vi "Get Value from JSON Text with Parameter.vi"(8 "error in (no error)":errorcluster, 10 "Parameter":string, 11 "JSON Configuration File (.json)":path=path "C:/Users/chericks/Desktop/JSONtest/labview-grpc-query-server/jsontestfile2.json") -> (0 "error out":errorcluster, 2 "Value":string="6")   [LabVIEW 2019]
panel:
  in  "Parameter List (for unit testing)":string[](array[string])=["GETCONF=SMUResourceName", "GETCONF=SMUChannels", "GETCONF=SMUSourceMode_Sequence", "GETCONF=SMUOutputFunction_DCCurrent", "GETCONF=SMUSourceTransientResponse_Fast", "GETCONF=SMUCurrent", "GETCONF=SMUCurrentLevelRange", "GETCONF=SMUMeasurementSense_Local", "GETCONF=SMUMeasurementApertureTime", "GETCONF=SMUSourceAdvancedSourceDelay", "GETCONF=SMUVoltage", "GETCONF=SMUSourceAdvancedSequenceLoopCount", "GETCONF=SMUMeasurementAdvancedDCNoiseRejection_Normal", "GETCONF=SMUSequenceName", "GETCONF=SMUStep1_Source_DCCurrent_CurrentLevel", "GETCONF=SMUStep2_Measurement_ApertureTime", "GETCONF=SMUStep3_Source_Advanced_SourceDelay", "GETCONF=SMUSequenceNumberOfSteps", "GETCONF=SMUTriggerFromSwitch_StartDigitalEdge", "GETCONF=SMUTriggerFromSwitch_SequenceAdvanceDigitalEdge", "GETCONF=SMUTriggerToDMM_SourceCompleteEvent", "GETCONF=SMUTriggerToDMM_SourceCompleteEvent_Value", "GETCONF=SMUTriggerToSwitch_SequenceIterationCompleteEvent", "GETCONF=SMUTriggerToDMM_SequenceIterationCompleteEvent_Value", "GETCONF=Switch1ResourceName", "GETCONF=Switch1Topology", "GETCONF=Switch1ScanList", "GETCONF=Switch2ResourceName", "GETCONF=Switch2Topology", "GETCONF=Switch2ScanList", "GETCONF=DMMResourceName", "GETCONF=DMMFunction_DCVolts", "GETCONF=DMMResolution", "GETCONF=DMMRange", "GETCONF=DMMTriggerSource_TTL2", "GETCONF=DMMTriggerSlope_RisingEdge", "GETCONF=DMMSampleTrigger_TTL2", "GETCONF=DMMSampleCount", "GETCONF=DMMSampleTriggerSlope_RisingEdge", "GETCONF=DMMApertureTimeUnits_Seconds", "GETCONF=DMMApertureTime", "GETCONF=DMMNumberOfAverages", "GETCONF=DMMAutoZero_Off", "GETCONF=DMMADCCalibration_Off", "GETCONF=DMMSettleTime", "GETCONF=DMMControlAction_Commit", "GETCONF=ApplicationNumberOfWeldChannels"]
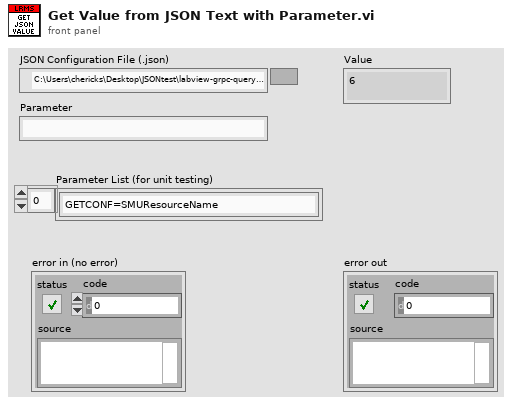
[diagram p1: front panel]
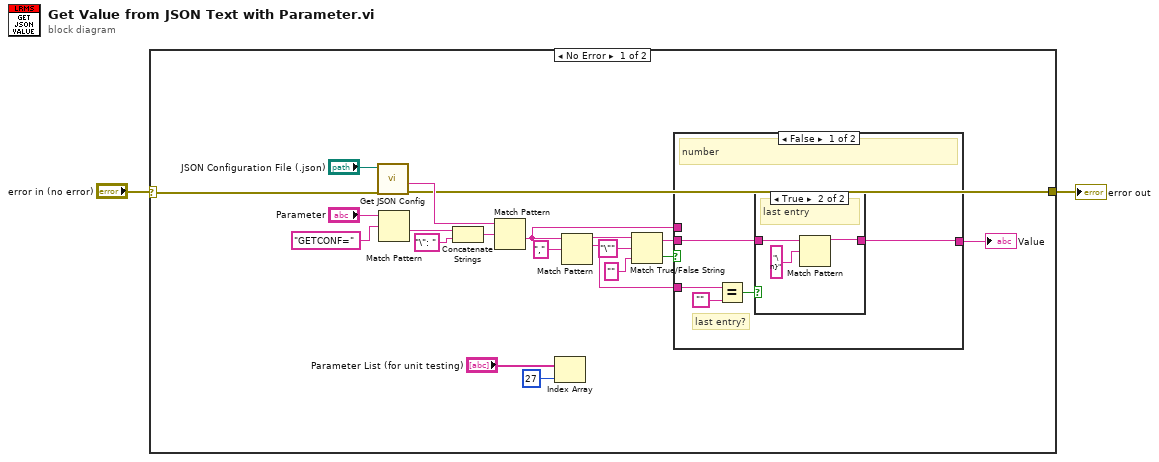
[diagram p0: block diagram]
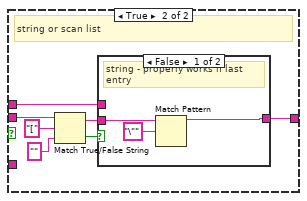
[diagram p3: hidden frame]
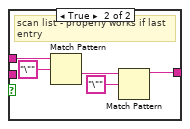
[diagram p4: hidden frame]
diagram:
  n1 = case shown="No Error" "error in (no error)" {
    selector: "error in (no error)" -> [w4 w47]
    tunnel: [w3 w47] -> w1
    frame No Error {
      n2 = call "Get JSON Config.vi"("error in (no error)"=w4, "JSON Configuration File (.json)"="JSON Configuration File (.json)") -> ("error out"=w3:errorcluster, "File Contents"=w5:string)  [unwired: 6 in, 2 out]
      n3 = Match Pattern(string="Parameter", regular expression="GETCONF=" ("default value 1")) -> (after substring=w10:string)  [unwired: 1 in, 3 out]
      n4 = Concatenate Strings(w10, "\": " ("string")) -> (w13:string)
      n5 = Match Pattern(string=w5, regular expression=w13) -> (after substring=w21:string)  [unwired: 1 in, 3 out]
      n6 = Index Array(array="Parameter List (for unit testing)", index=27) -> ()  [unwired: 1 out]
      n7 = Match Pattern(string=w21, regular expression=",") -> (before substring=w17:string, match substring=w19:string)  [unwired: 1 in, 2 out]
      n8 = Match True/False String(2:"" ("false string"), 3:"\"" ("true string"), 4:w17) -> (0:w18:bool, 1:w20:string)
      n9 = case shown="False" w18 {
        tunnel: [w23 w34] -> w9
        tunnel: w19 -> [w26 _]
        tunnel: w20 -> [w24 w38]
        tunnel: w21 -> [_ w33]
        frame False {
          # "last entry?"
          # "number"
          n10 = Equal?(x=w26, y="") -> (x = y?=w25:bool)
          n11 = case shown="True" w25 {
            tunnel: w24 -> [w28 w31]
            tunnel: [w28 w29] -> w23
            frame False {
              # "not last entry"
            }
            frame True {
              # "last entry"
              n12 = Match Pattern(string=w31, regular expression="\n}" ("string")) -> (before substring=w29:string)  [unwired: 1 in, 3 out]
            }
          }
        }
        frame True {
          # "string or scan list"
          n13 = Match True/False String(2:"" ("false string"), 3:"[" ("true string"), 4:w38) -> (0:w35:bool, 1:w32:string)
          n14 = case shown="False" w35 {
            tunnel: [w39 w42] -> w34
            tunnel: w33 -> [_ w46]
            tunnel: w32 -> [w41 _]
            frame False {
              # "string - properly works if last entry"
              n15 = Match Pattern(string=w41, regular expression="\"") -> (before substring=w39:string)  [unwired: 1 in, 3 out]
            }
            frame True {
              # "scan list - properly works if last entry"
              n16 = Match Pattern(string=w46, regular expression="\"") -> (after substring=w44:string)  [unwired: 1 in, 3 out]
              n17 = Match Pattern(string=w44, regular expression="\"") -> (before substring=w42:string)  [unwired: 1 in, 3 out]
            }
          }
        }
      }
      "Value" <- w9
    }
    frame Error {
    }
  }
  "error out" <- w1
